vi "modify.vi"(8 "error in (no error)":errorcluster, 11 "StringGeneratorAK110125StimServerCmd in":refnum<class "StringGeneratorAK110125StimServerCmd.lvclass">) -> (0 "error out":errorcluster, 2 "string":string, 3 "StringGeneratorAK110125StimServerCmd out":refnum<class "StringGeneratorAK110125StimServerCmd.lvclass">)   [LabVIEW 2010, in "StringGeneratorAK110125StimServerCmd.lvclass"]
uses:
  StringGeneratorAK110125StimServerCmd.lvclass
  StringGeneratorAK110125StimServerCmd.lvclass/StringGeneratorAK110125StimServerCmd.ctl
panel:
  in  "save":bool
  in  "load":bool
  in  "stimulus":string
  in  "cancel":bool
  in  "ok":bool
  in  "sequence IDs with spaces":string
  in  "settings":string(combo)
  in  "blank time (s)":string="1"
  in  "randomize":bool
  in  "user sequence":bool
  # "StringGeneratorAK110125StimServerCmd"
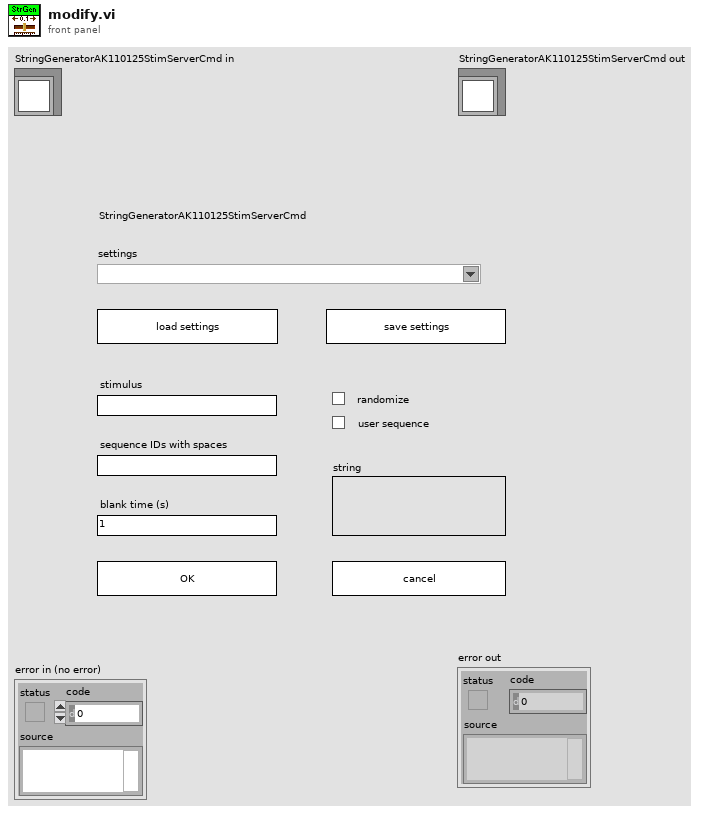
[diagram p1: front panel]
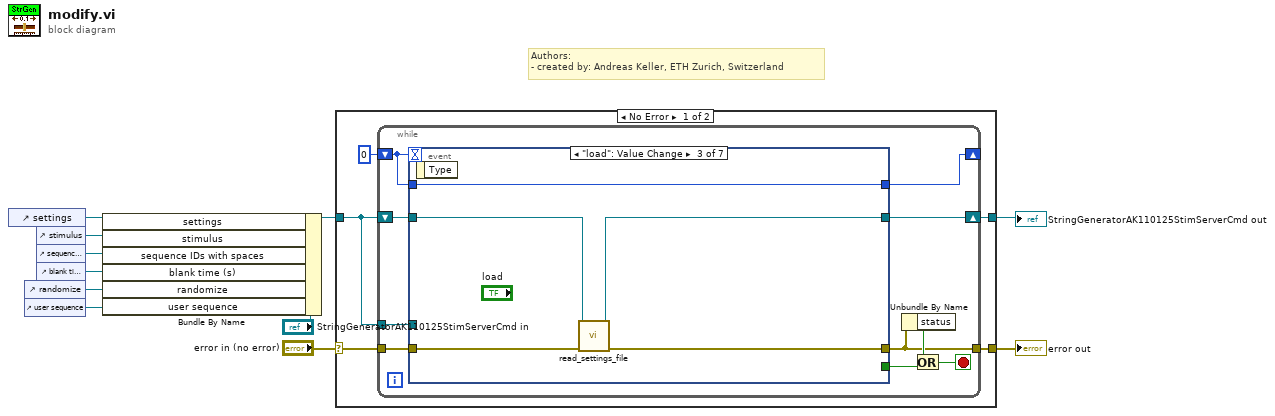
[diagram p0: block diagram]
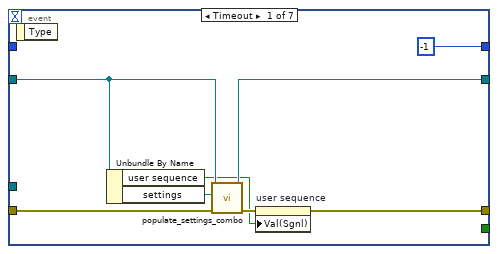
[diagram p2: hidden frame]
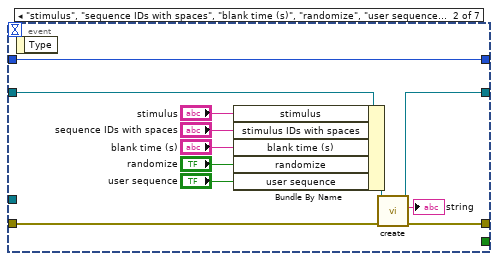
[diagram p3: hidden frame]
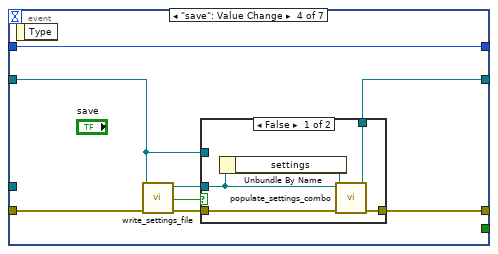
[diagram p4: hidden frame]
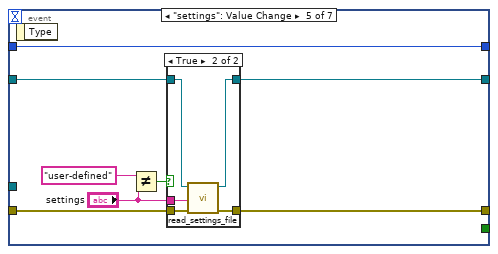
[diagram p6: hidden frame]
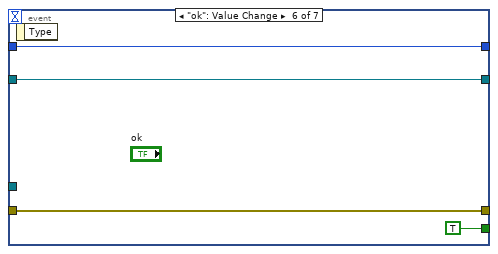
[diagram p8: hidden frame]
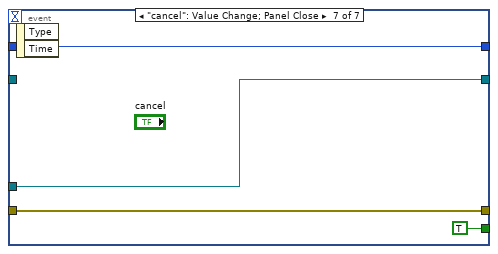
[diagram p9: hidden frame]
diagram:
  # "Authors: \n- created by: Andreas Keller, ETH Zurich, Switzerland"
  n1 = control-ref of="settings"() -> (w4:refnum<vi>)
  n2 = control-ref of="randomize"() -> (w5:refnum<vi>)
  n3 = control-ref of="user sequence"() -> (w6:refnum<vi>)
  n4 = control-ref of="stimulus"() -> (w9:refnum<vi>)
  n5 = control-ref of="sequence IDs with spaces"() -> (w8:refnum<vi>)
  n6 = control-ref of="blank time (s)"() -> (w7:refnum<vi>)
  n7 = Bundle By Name(cluster="StringGeneratorAK110125StimServerCmd in", "settings"=w4, "stimulus"=w9, "sequence IDs with spaces"=w8, "blank time (s)"=w7, "randomize"=w5, "user sequence"=w6) -> (w3:refnum<class "StringGeneratorAK110125StimServerCmd.lvclass">)
  n8 = case shown="No Error" "error in (no error)" {
    selector: "error in (no error)" -> [w15 w90]
    tunnel: [w16 w90] -> w11
    tunnel: w3 -> [w12 w91]
    tunnel: [w14 w91] -> w10
    frame No Error {
      n9 = while {
        tunnel: [w20] -> w16
        tunnel: w15 -> [w25]
        shift-right: [w22] -> _
        shift-left: 0 -> [w23]
        tunnel: w12 -> [w17]
        shift-right: [w24] -> w14
        shift-left: w12 -> [w26]
        stop <- w18 stop-if-true
        n10 = event shown="[2] \"load\": Value Change" {
          selector: _ -> [_ _ _ _ _ _ _]
          dyn-events: _ -> [_ _ _ _ _ _ _]
          timeout: w23 -> [_ _ _ _ _ _ _]
          tunnel: w26 -> [w31 w45 w48 w56 w68 w83 _]
          tunnel: [w28 w40 w49 w57 w69 w82 w89] -> w20
          tunnel: w25 -> [w32 w41 w50 w55 w70 w82 w89]
          tunnel: [w30 w42 w47 w58 w67 w83 w86] -> w24
          tunnel: w23 -> [_ w46 w51 w59 w74 w85 w88]
          tunnel: [-1 w46 w51 w59 w74 w85 w88] -> w22
          tunnel: [_ _ _ _ _ TRUE TRUE] -> w19
          tunnel: w17 -> [_ _ _ _ _ _ w86]
          event Timeout {
            n11 = event-data() -> ()  [unwired: 1 in, 1 out]
            n12 = Unbundle By Name(w31) -> ("user sequence"=w27:bool, "settings"=w33:refnum<vi>)
            n13 = call-dynamic "populate_settings_combo.vi"("error in (no error)"=w32, "combo box ref"=w33, "GenericPlugin in"=w31) -> ("error out"=w29:errorcluster, "GenericPlugin out"=w30:refnum<class "StringGeneratorAK110125StimServerCmd.lvclass">)  [unwired: 7 in]
            n14 = property on="user sequence" class="Bool (strict)"(error in=w29, "Val(Sgnl)"=w27) -> (error out=w28:errorcluster)  [unwired: 1 in, 1 out]
          }
          event "stimulus", "sequence IDs with spaces", "blank time (s)", "randomize", "user sequence": Value Change {
            n15 = event-data() -> ()  [unwired: 1 in, 1 out]
            n16 = Bundle By Name(cluster=w45, "stimulus"="stimulus", "stimulus IDs with spaces"="sequence IDs with spaces", "blank time (s)"="blank time (s)", "randomize"="randomize", "user sequence"="user sequence") -> (w43:refnum<class "StringGeneratorAK110125StimServerCmd.lvclass">)
            n17 = call-dynamic "create.vi"("error in (no error)"=w41, "StringGeneratorAK110125StimServerCmd in"=w43) -> ("error out"=w40:errorcluster, "string"=→"string":string, "StringGeneratorAK110125StimServerCmd out"=w42:refnum<class "StringGeneratorAK110125StimServerCmd.lvclass">)  [unwired: 7 in]
          }
          event "load": Value Change {
            n18 = event-data() -> ()  [unwired: 1 in, 1 out]
            n19 = call-dynamic "read_settings_file.vi"("error in (no error)"=w50, "GenericPlugin in"=w48) -> ("error out"=w49:errorcluster, "GenericPlugin out"=w47:refnum<class "StringGeneratorAK110125StimServerCmd.lvclass">)  [unwired: 7 in, 1 out]
          }
          event "save": Value Change {
            n20 = event-data() -> ()  [unwired: 1 in, 1 out]
            n21 = call-dynamic "write_settings_file.vi"("error in (no error)"=w55, "GenericPlugin in"=w56) -> ("error out"=w54:errorcluster, "cancelled?"=w53:bool, "GenericPlugin out"=w52:refnum<class "StringGeneratorAK110125StimServerCmd.lvclass">)  [unwired: 6 in, 1 out]
            n22 = case shown="False" w53 {
              tunnel: w52 -> [w63 _]
              tunnel: [w62 w66] -> w58
              tunnel: w54 -> [w61 w65]
              tunnel: [w60 w65] -> w57
              tunnel: w56 -> [_ w66]
              frame False {
                n23 = Unbundle By Name(w63) -> ("settings"=w64:refnum<vi>)
                n24 = call-dynamic "populate_settings_combo.vi"("error in (no error)"=w61, "combo box ref"=w64, "GenericPlugin in"=w63) -> ("error out"=w60:errorcluster, "GenericPlugin out"=w62:refnum<class "StringGeneratorAK110125StimServerCmd.lvclass">)  [unwired: 7 in]
              }
              frame True {
              }
            }
          }
          event "settings": Value Change {
            n25 = event-data() -> ()  [unwired: 1 in, 1 out]
            n26 = Not Equal?(x="user-defined", y="settings") -> (x != y?=w72:bool)
            n27 = case shown="True" w72 {
              tunnel: "settings" -> [_ w81]
              tunnel: w70 -> [w75 w80]
              tunnel: [w75 w79] -> w69
              tunnel: w68 -> [w76 w78]
              tunnel: [w76 w77] -> w67
              frame False {
              }
              frame True {
                n28 = call-dynamic "read_settings_file.vi"("error in (no error)"=w80, "settings name"=w81, "GenericPlugin in"=w78) -> ("error out"=w79:errorcluster, "GenericPlugin out"=w77:refnum<class "StringGeneratorAK110125StimServerCmd.lvclass">)  [unwired: 6 in, 1 out]
              }
            }
          }
          event "ok": Value Change {
            n29 = event-data() -> ()  [unwired: 1 in, 1 out]
          }
          event "cancel": Value Change; Panel Close {
            n30 = event-data() -> ()  [unwired: 1 in, 2 out]
          }
        }
        n31 = Unbundle By Name(w20) -> ("status"=w21:bool)
        n32 = Or(x=w21, y=w19) -> (x .or. y?=w18:bool)
      }
    }
    frame Error {
    }
  }
  "error out" <- w11
  "StringGeneratorAK110125StimServerCmd out" <- w10
